vi "N08_Cluster.vi"() -> ()   [LabVIEW 2023]
panel:
  in  "Cluster 2":T1
  out "Numeric B Name":dbl
  out "String":string
  out "Boolean":bool
  out "Numeric A":dbl
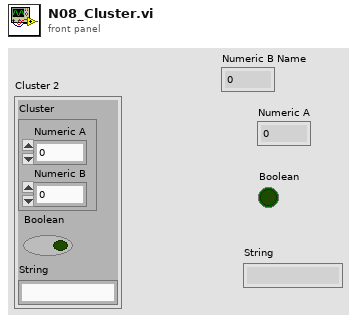
[diagram p1: front panel]
types:
  T1 = cluster{"Cluster":cluster{"Numeric A":dbl, "Numeric B":dbl}, "Boolean":bool, "String":string}
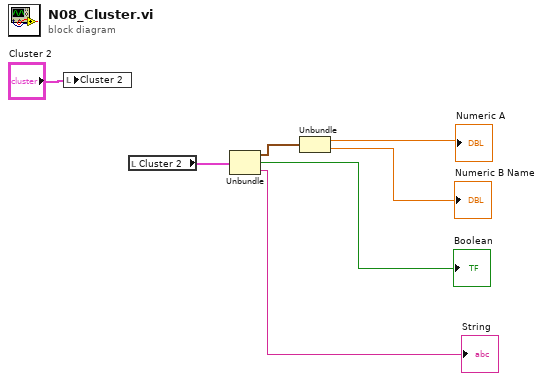
[diagram p0: block diagram]
diagram:
  n1 = local write "Cluster 2"("Cluster 2") -> ()
  n2 = local read "Cluster 2"() -> (w6:T1)
  n3 = Unbundle(w6) -> ("Cluster"=w5:cluster{"Numeric A":dbl, "Numeric B":dbl}, "Boolean"=→"Boolean":bool, "String"=→"String":string)
  n4 = Unbundle(w5) -> ("Numeric A"=→"Numeric A":dbl, "Numeric B"=→"Numeric B Name":dbl)
